vi "ARC_Comm Get Next Event.vi"(4 "Error Handle":string="UI:Core - Error", 6 "error in (no error)":errorcluster, 7 "event queue in":string[](array[string])) -> (0 "prev event":string, 1 "next event":string, 2 "event queue out":string[](array[string]))   [LabVIEW 2016]
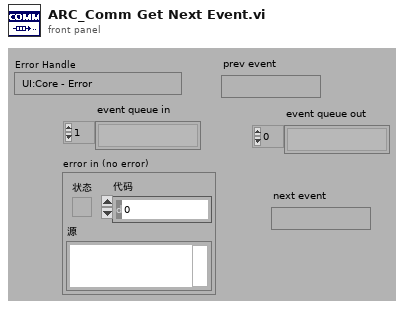
[diagram p1: front panel]
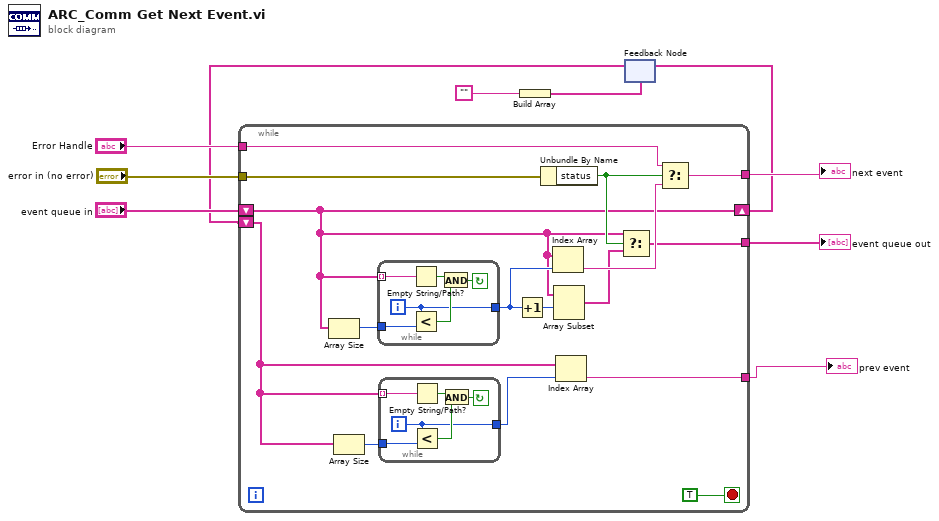
[diagram p0: block diagram]
diagram:
  n1 = Build Array("") -> (w5:string[])
  n2 = feedback #1(w5) -> (w2:string[])
  n3 = while {
    tunnel: "Error Handle" -> [w23]
    tunnel: [w21] -> w9
    tunnel: "error in (no error)" -> [w20]
    tunnel: [w18] -> w7
    tunnel: [w13] -> w1
    shift-right: [w12] -> w3
    shift-left: "event queue in" -> [w12]
    shift-left: w2 -> [w11]
    stop <- TRUE stop-if-true
    n4 = Array Size(array=w12) -> (size(s)=w25:i32)
    n5 = Array Size(array=w11) -> (size(s)=w15:i32)
    n6 = while {
      tunnel: w12 -> [w38] mode=indexing
      tunnel: w25 -> [w37]
      tunnel: [w33] -> w24
      i -> [w33]
      stop <- w34 continue-if-true
      n7 = Empty String/Path?(string/path=w38) -> (empty?=w36:bool)
      n8 = Less?(x=w33, y=w37) -> (x < y?=w35:bool)
      n9 = And(x=w36, y=w35) -> (x .and. y?=w34:bool)
    }
    n10 = while {
      tunnel: w11 -> [w32] mode=indexing
      tunnel: w15 -> [w31]
      tunnel: [w27] -> w14
      i -> [w27]
      stop <- w28 continue-if-true
      n11 = Empty String/Path?(string/path=w32) -> (empty?=w30:bool)
      n12 = Less?(x=w27, y=w31) -> (x < y?=w29:bool)
      n13 = And(x=w30, y=w29) -> (x .and. y?=w28:bool)
    }
    n14 = Increment(x=w24) -> (x+1=w26:i32)
    n15 = Unbundle By Name(w20) -> ("status"=w19:bool)
    n16 = Index Array(array=w12, index=w24) -> (element=w22:string)
    n17 = Array Subset(array=w12, index=w26) -> (w17:string[])  [unwired: 1 in]
    n18 = Index Array(array=w11, index=w14) -> (element=w13:string)
    n19 = Select(t=w12, s=w19, f=w17) -> (s? t:f=w18:string[])
    n20 = Select(t=w23, s=w19, f=w22) -> (s? t:f=w21:string)
  }
  "event queue out" <- w7
  "next event" <- w9
  "prev event" <- w1
  n21 = feedback-in #1(w3) -> ()
